vi "SaveData_Roberto.vi"(2 "Quad sub area":dbl format="%#_13g", 4 "Ext time (sec)":dbl=3598463718.5222077 format="%#_10g", 6 "Array":dbl[](array[numeric])=[213.0, 0.002, 401.0, 60.0, 24.0, 3.279, 1.868, 1.4806, 8.203, -0.16493333333333543, 1.0, 1000.0, 1.0, 1.0, 0.0, 0.0101, 0.0101, 0.0101, 0.0099, 0.0101, 0.0099, 0.0099, 0.0099, 0.0099, 0.0098, 0.0098, 0.0098, 0.0096, 0.0096, 0.0096, 0.0095, 0.0095, 0.0095, 0.0093, 0.0093, 0.0093, 0.0093, 0.0092, 0.0092, 0.0092, 0.0092, 0.009, 0.0092, 0.009, 0.009, 0.0089, 0.0089, 0.0089, 0.0089, 0.0087, 0.0087, 0.0087, 0.0087, 0.0087, 0.0085, 0.0087, 0.0085, 0.0084, 0.0085, 0.0085, 0.0084, 0.0082, 0.0082, 0.0082, 0.0081, 0.0081, 0.0081, 0.0081, 0.0081, 0.0081, 0.0079, 0.0079, 0.0079, 0.0079, 0.0078, 0.0078, 0.0076, 0.0076, 0.0076, 0.0078, 0.0078, 0.0078, 0.0076, 0.0075, 0.0075, 0.0075, 0.0073, 0.0075, 0.0075, 0.0073, 0.0073, 0.0073, 0.0072, 0.0072, 0.0072, 0.0072, 0.0072, 0.007, 0.0072, 0.0072, 0.0072, 0.0072, 0.007, 0.007, 0.007, 0.007, 0.0069, 0.0069, 0.0069, 0.007, 0.0069, 0.0069, 0.0067, 0.0069, 0.0069, 0.0067, 0.0067, 0.0069, 0.0067, 0.0066, 0.0066, 0.0066, 0.0066, 0.0067, 0.0066, 0.0066, 0.0066, 0.0066, 0.0066, 0.0066, 0.0064, 0.0064, 0.0064, 0.0066, 0.0064, 0.0064, 0.0066, 0.0064, 0.0064, 0.0064, 0.0066, 0.0066, 0.0064, 0.0064, 0.0064, 0.0064, 0.0064, 0.0064, 0.0064, 0.0064, 0.0066, 0.0066, 0.0064, 0.0066, 0.0066, 0.0066, 0.0066, 0.0066, 0.0066, 0.0064, 0.0067, 0.0067, 0.0067, 0.0069, 0.0069, 0.0069, 0.0072, 0.0072, 0.0073, 0.0073, 0.0073, 0.0075, 0.0076, 0.0078, 0.0079, 0.0082, 0.0084, 0.0087, 0.009, 0.0093, 0.0095, 0.0098, 0.0104, 0.0107, 0.0111, 0.0114, 0.0117, 0.0121, 0.0122, 0.0122, 0.0122, 0.0124, 0.0121, 0.0117, 0.0114, 0.011, 0.0107, 0.0104, 0.0101, 0.0098, 0.0093, 0.0093, 0.0092, 0.009, 0.0089, 0.0089, 0.0089, 0.0087, 0.0085, 0.0085, 0.0085, 0.0084, 0.0085, 0.0082, 0.0081, 0.0081, 0.0079, 0.0079, 0.0079, 0.0078, 0.0079, 0.0079, 0.0079, 0.0079, 0.0079, 0.0081, 0.0082, 0.0082, 0.0082, 0.0085, 0.0084, 0.0084, 0.0085, 0.0082, 0.0082, 0.0082, 0.0081, 0.0079, 0.0078, 0.0076, 0.0075, 0.0073, 0.0072, 0.007, 0.007, 0.007, 0.0072, 0.007, 0.0072, 0.007, 0.007, 0.007, 0.0069, 0.007, 0.0069, 0.007, 0.007, 0.007, 0.007, 0.0069, 0.0069, 0.0069, 0.0069, 0.0067, 0.0067, 0.0067, 0.0067, 0.0066, 0.0066, 0.0067, 0.0064, 0.0064, 0.0066, 0.0066, 0.0066, 0.0067, 0.0067, 0.0067, 0.0066, 0.0069, 0.0069, 0.0069, 0.0067, 0.0069, 0.0069, 0.007, 0.007, 0.007, 0.007, 0.007, 0.0072, 0.0072, 0.0072, 0.0073, 0.0072, 0.0073, 0.0073, 0.0072, 0.0073, 0.0072, 0.0072, 0.007, 0.0072, 0.0072, 0.0072, 0.0072, 0.0072, 0.0072, 0.007, 0.007, 0.007, 0.0072, 0.0072, 0.0072, 0.0073, 0.0072, 0.0072, 0.0072, 0.0072, 0.0073, 0.0073, 0.0072, 0.0073, 0.0073, 0.0073, 0.0073, 0.0073, 0.0073, 0.0073, 0.0073, 0.0075, 0.0075, 0.0075, 0.0075, 0.0076, 0.0078, 0.0075, 0.0076, 0.0078, 0.0078, 0.0078, 0.0078, 0.0078, 0.0078, 0.0078, 0.0078, 0.0079, 0.0079, 0.0079, 0.0079, 0.0079, 0.0081, 0.0082, 0.0081, 0.0084, 0.0084, 0.0084, 0.0084, 0.0085, 0.0084, 0.0085, 0.0085, 0.0087, 0.0087, 0.0089, 0.0089, 0.0089, 0.0089, 0.0089, 0.0089, 0.009, 0.009, 0.0092, 0.009, 0.0092, 0.0092, 0.0093, 0.0093, 0.0095, 0.0095, 0.0095, 0.0095, 0.0096, 0.0096, 0.0098, 0.0098, 0.0099, 0.0099, 0.0101, 0.0101, 0.0101, 0.0101, 0.0101, 0.0102, 0.0102, 0.0102, 0.0102, 0.0104, 0.0104, 0.0104, 0.0107, 0.0105, 0.0107, 0.0108, 0.0108, 0.0108, 0.0108, 0.011, 0.0111, 0.0111, 0.011, 0.0111, 0.0111, 0.0111, 0.0111, 0.0111]) -> (0 "Frequency":dbl=212.9519, 1 "Area":dbl=0.0007273210385932467 format="%#_5g", 3 "Current time (sec)":dbl=3598463780.505753 format="%#_10g", 5 "ADC value":dbl[](array[numeric])=[0.0, 0.0, 0.0, 0.0, 0.0, 0.0, 0.0, 0.0, 0.0, 0.0, 0.0, 0.0, 0.0, 0.0, 0.0, 0.0, 0.0, 0.0, 0.0, 0.0, 0.0, 0.0, 0.0, 0.0, 0.0, 0.0, -0.0, 0.0, 0.0, 0.0, 0.0, -0.0, -0.0, 0.0, 0.0, 0.0, -0.0, 0.0, 0.0, 0.0, 0.0, -0.0, -0.0001, 0.0, 0.0, -0.0, -0.0, -0.0, -0.0, -0.0, -0.0001, -0.0, -0.0, -0.0, 0.0, 0.0, 0.0, 0.0, 0.0, -0.0, -0.0, -0.0, -0.0, -0.0, 0.0, 0.0, 0.0, 0.0, 0.0, -0.0, -0.0, -0.0, 0.0, -0.0, -0.0, -0.0, 0.0, -0.0, -0.0, 0.0, 0.0, 0.0001, 0.0001, 0.0001, 0.0001, 0.0, 0.0001, 0.0, 0.0001, 0.0001, 0.0001, 0.0001, 0.0001, 0.0001, 0.0001, 0.0001, 0.0001, 0.0001, 0.0001, 0.0001, 0.0001, 0.0001, 0.0001, 0.0001, 0.0001, 0.0001, 0.0001, 0.0001, 0.0001, 0.0002, 0.0001, 0.0002, 0.0002, 0.0002, 0.0002, 0.0002, 0.0002, 0.0001, 0.0002, 0.0002, 0.0002, 0.0003, 0.0003, 0.0003, 0.0002, 0.0004, 0.0003, 0.0003, 0.0003, 0.0003, 0.0003, 0.0004, 0.0004, 0.0004, 0.0004, 0.0005, 0.0005, 0.0005, 0.0005, 0.0006, 0.0006, 0.0007, 0.0007, 0.0007, 0.0007, 0.0008, 0.0008, 0.0009, 0.0009, 0.001, 0.0011, 0.0011, 0.0012, 0.0013, 0.0013, 0.0014, 0.0016, 0.0017, 0.0018, 0.0019, 0.0021, 0.0023, 0.0025, 0.0027, 0.0029, 0.0032, 0.0035, 0.0038, 0.0041, 0.0044, 0.0047, 0.005, 0.0052, 0.0053, 0.0054, 0.0054, 0.0053, 0.0052, 0.0049, 0.0047, 0.0044, 0.0041, 0.0038, 0.0036, 0.0034, 0.0031, 0.003, 0.0029, 0.0028, 0.0027, 0.0027, 0.0026, 0.0026, 0.0025, 0.0025, 0.0024, 0.0023, 0.0023, 0.0022, 0.0022, 0.0021, 0.002, 0.002, 0.0019, 0.002, 0.0019, 0.002, 0.002, 0.0021, 0.0021, 0.0021, 0.0023, 0.0023, 0.0023, 0.0024, 0.0024, 0.0024, 0.0024, 0.0023, 0.0022, 0.0022, 0.0021, 0.0019, 0.0018, 0.0017, 0.0016, 0.0015, 0.0014, 0.0013, 0.0013, 0.0013, 0.0012, 0.0012, 0.0012, 0.0012, 0.0012, 0.0012, 0.0011, 0.0011, 0.0011, 0.0012, 0.0011, 0.0011, 0.0011, 0.0011, 0.001, 0.001, 0.001, 0.0009, 0.0008, 0.0008, 0.0007, 0.0007, 0.0006, 0.0007, 0.0006, 0.0006, 0.0006, 0.0006, 0.0006, 0.0005, 0.0005, 0.0006, 0.0006, 0.0006, 0.0006, 0.0006, 0.0006, 0.0007, 0.0007, 0.0007, 0.0007, 0.0007, 0.0007, 0.0007, 0.0008, 0.0008, 0.0008, 0.0008, 0.0008, 0.0008, 0.0007, 0.0007, 0.0007, 0.0006, 0.0006, 0.0006, 0.0006, 0.0005, 0.0005, 0.0004, 0.0005, 0.0004, 0.0003, 0.0003, 0.0003, 0.0003, 0.0003, 0.0003, 0.0003, 0.0003, 0.0003, 0.0003, 0.0002, 0.0002, 0.0002, 0.0002, 0.0002, 0.0002, 0.0001, 0.0001, 0.0001, 0.0002, 0.0001, 0.0001, 0.0001, 0.0001, 0.0, 0.0, -0.0, 0.0001, -0.0, -0.0, 0.0, -0.0, -0.0001, -0.0, -0.0001, -0.0001, -0.0001, -0.0002, -0.0001, -0.0001, -0.0001, -0.0001, -0.0001, -0.0001, -0.0001, -0.0001, -0.0001, -0.0, -0.0, -0.0001, -0.0, -0.0, -0.0, 0.0, 0.0001, 0.0, 0.0, 0.0001, 0.0001, 0.0, 0.0, 0.0, -0.0, -0.0, -0.0, -0.0001, -0.0, -0.0, -0.0, -0.0001, -0.0, -0.0, -0.0, -0.0, -0.0, 0.0, 0.0, 0.0, 0.0, 0.0001, 0.0, 0.0, 0.0, 0.0, 0.0, 0.0, 0.0, 0.0, 0.0, 0.0, 0.0, 0.0, 0.0, 0.0, 0.0, 0.0, 0.0, 0.0, 0.0, 0.0, 0.0, 0.0, 0.0, 0.0, 0.0, 0.0, 0.0, 0.0])   [LabVIEW 2018]
uses:
  Global 2.vi
  kleinjan/MKS/Global - Pressure & Flow.vi
  <vilib>/Utility/file.llb/Write To Spreadsheet File (string).vi
  <vilib>/Utility/file.llb/Write To Spreadsheet File (DBL).vi
panel:
  out "Fit OK":bool=TRUE
  out "Fupper":dbl=213.3 format="%#_13g"
  out "Flower":dbl=212.75 format="%#_13g"
  out "Python data":i32=2914
  out "String to python":string="213 MHz crystal, SMT03 RF Gen\r\nQCV3598374279.csv\r\nUnused\r\nNMRave.csv\r\nUnused\r\nTune2.csv\r\n\r\n\r\n  212.7500\r\n  213.3000\r\n35984.0000\r\n63780.5058\r\n  213.0000\r\n    0.0020\r\n  401.0000\r\n   60.0000\r\n   24.0000\r\n    3.2790\r\n    1.8680\r\n    1.4806\r\n    8.2030\r\n   -0.1649\r\n    1.0000\r\n 1000.0000\r\n    1.0000\r\n    1.0000\r\n    0.0000\r\n    4.0771\r\n    2.0000\r\n  212.9500\r\n    0.0000\r\n    0.0000\r\n    4.0000\r\n    2.1333\r\n   33.8900\r\n    0.0101\r\n    0.0101\r\n    0.0101\r\n    0.0099\r\n    0.0101\r\n    0.0099\r\n    0.0099\r\n    0.0099\r\n    0.0099\r\n    0.0098\r\n    0.0098\r\n    0.0098\r\n    0.0096\r\n    0.0096\r\n    0.0096\r\n    0.0095\r\n    0.0095\r\n    0.0095\r\n    0.0093\r\n    0.0093\r\n    0.0093\r\n    0.0093\r\n    0.0092\r\n    0.0092\r\n    0.0092\r\n    0.0092\r\n    0.0090\r\n    0.0092\r\n    0.0090\r\n    0.0090\r\n    0.0089\r\n    0.0089\r\n    0.0089\r\n    0.0089\r\n    0.0087\r\n    0.0087\r\n    0.0087\r\n    0.0087\r\n    0.0087\r\n    0.0085\r\n    0.0087\r\n    0.0085\r\n    0.0084\r\n    0.0085\r\n    0.0085\r\n    0.0084\r\n    0.0082\r\n    0.0082\r\n    0.0082\r\n    0.0081\r\n    0.0081\r\n    0.0081\r\n    0.0081\r\n    0.0081\r\n    0.0081\r\n    0.0079\r\n    0.0079\r\n    0.0079\r\n    0.0079\r\n    0.0078\r\n    0.0078\r\n    0.0076\r\n    0.0076\r\n    0.0076\r\n    0.0078\r\n    0.0078\r\n    0.0078\r\n    0.0076\r\n    0.0075\r\n    0.0075\r\n    0.0075\r\n    0.0073\r\n    0.0075\r\n    0.0075\r\n    0.0073\r\n    0.0073\r\n    0.0073\r\n    0.0072\r\n    0.0072\r\n    0.0072\r\n    0.0072\r\n    0.0072\r\n    0.0070\r\n    0.0072\r\n    0.0072\r\n    0.0072\r\n    0.0072\r\n    0.0070\r\n    0.0070\r\n    0.0070\r\n    0.0070\r\n    0.0069\r\n    0.0069\r\n    0.0069\r\n    0.0070\r\n    0.0069\r\n    0.0069\r\n    0.0067\r\n    0.0069\r\n    0.0069\r\n    0.0067\r\n    0.0067\r\n    0.0069\r\n    0.0067\r\n    0.0066\r\n    0.0066\r\n    0.0066\r\n    0.0066\r\n    0.0067\r\n    0.0066\r\n    0.0066\r\n    0.0066\r\n    0.0066\r\n    0.0066\r\n    0.0066\r\n    0.0064\r\n    0.0064\r\n    0.0064\r\n    0.0066\r\n    0.0064\r\n    0.0064\r\n    0.0066\r\n    0.0064\r\n    0.0064\r\n    0.0064\r\n    0.0066\r\n    0.0066\r\n    0.0064\r\n    0.0064\r\n    0.0064\r\n    0.0064\r\n    0.0064\r\n    0.0064\r\n    0.0064\r\n    0.0064\r\n    0.0066\r\n    0.0066\r\n    0.0064\r\n    0.0066\r\n    0.0066\r\n    0.0066\r\n    0.0066\r\n    0.0066\r\n    0.0066\r\n    0.0064\r\n    0.0067\r\n    0.0067\r\n    0.0067\r\n    0.0069\r\n    0.0069\r\n    0.0069\r\n    0.0072\r\n    0.0072\r\n    0.0073\r\n    0.0073\r\n    0.0073\r\n    0.0075\r\n    0.0076\r\n    0.0078\r\n    0.0079\r\n    0.0082\r\n    0.0084\r\n    0.0087\r\n    0.0090\r\n    0.0093\r\n    0.0095\r\n    0.0098\r\n    0.0104\r\n    0.0107\r\n    0.0111\r\n    0.0114\r\n    0.0117\r\n    0.0121\r\n    0.0122\r\n    0.0122\r\n    0.0122\r\n    0.0124\r\n    0.0121\r\n    0.0117\r\n    0.0114\r\n    0.0110\r\n    0.0107\r\n    0.0104\r\n    0.0101\r\n    0.0098\r\n    0.0093\r\n    0.0093\r\n    0.0092\r\n    0.0090\r\n    0.0089\r\n    0.0089\r\n    0.0089\r\n    0.0087\r\n    0.0085\r\n    0.0085\r\n    0.0085\r\n    0.0084\r\n    0.0085\r\n    0.0082\r\n    0.0081\r\n    0.0081\r\n    0.0079\r\n    0.0079\r\n    0.0079\r\n    0.0078\r\n    0.0079\r\n    0.0079\r\n    0.0079\r\n    0.0079\r\n    0.0079\r\n    0.0081\r\n    0.0082\r\n    0.0082\r\n    0.0082\r\n    0.0085\r\n    0.0084\r\n    0.0084\r\n    0.0085\r\n    0.0082\r\n    0.0082\r\n    0.0082\r\n    0.0081\r\n    0.0079\r\n    0.0078\r\n    0.0076\r\n    0.0075\r\n    0.0073\r\n    0.0072\r\n    0.0070\r\n    0.0070\r\n    0.0070\r\n    0.0072\r\n    0.0070\r\n    0.0072\r\n    0.0070\r\n    0.0070\r\n    0.0070\r\n    0.0069\r\n    0.0070\r\n    0.0069\r\n    0.0070\r\n    0.0070\r\n    0.0070\r\n    0.0070\r\n    0.0069\r\n    0.0069\r\n    0.0069\r\n    0.0069\r\n    0.0067\r\n    0.0067\r\n    0.0067\r\n    0.0067\r\n    0.0066\r\n    0.0066\r\n    0.0067\r\n    0.0064\r\n    0.0064\r\n    0.0066\r\n    0.0066\r\n    0.0066\r\n    0.0067\r\n    0.0067\r\n    0.0067\r\n    0.0066\r\n    0.0069\r\n    0.0069\r\n    0.0069\r\n    0.0067\r\n    0.0069\r\n    0.0069\r\n    0.0070\r\n    0.0070\r\n    0.0070\r\n    0.0070\r\n    0.0070\r\n    0.0072\r\n    0.0072\r\n    0.0072\r\n    0.0073\r\n    0.0072\r\n    0.0073\r\n    0.0073\r\n    0.0072\r\n    0.0073\r\n    0.0072\r\n    0.0072\r\n    0.0070\r\n    0.0072\r\n    0.0072\r\n    0.0072\r\n    0.0072\r\n    0.0072\r\n    0.0072\r\n    0.0070\r\n    0.0070\r\n    0.0070\r\n    0.0072\r\n    0.0072\r\n    0.0072\r\n    0.0073\r\n    0.0072\r\n    0.0072\r\n    0.0072\r\n    0.0072\r\n    0.0073\r\n    0.0073\r\n    0.0072\r\n    0.0073\r\n    0.0073\r\n    0.0073\r\n    0.0073\r\n    0.0073\r\n    0.0073\r\n    0.0073\r\n    0.0073\r\n    0.0075\r\n    0.0075\r\n    0.0075\r\n    0.0075\r\n    0.0076\r\n    0.0078\r\n    0.0075\r\n    0.0076\r\n    0.0078\r\n    0.0078\r\n    0.0078\r\n    0.0078\r\n    0.0078\r\n    0.0078\r\n    0.0078\r\n    0.0078\r\n    0.0079\r\n    0.0079\r\n    0.0079\r\n    0.0079\r\n    0.0079\r\n    0.0081\r\n    0.0082\r\n    0.0081\r\n    0.0084\r\n    0.0084\r\n    0.0084\r\n    0.0084\r\n    0.0085\r\n    0.0084\r\n    0.0085\r\n    0.0085\r\n    0.0087\r\n    0.0087\r\n    0.0089\r\n    0.0089\r\n    0.0089\r\n    0.0089\r\n    0.0089\r\n    0.0089\r\n    0.0090\r\n    0.0090\r\n    0.0092\r\n    0.0090\r\n    0.0092\r\n    0.0092\r\n    0.0093\r\n    0.0093\r\n    0.0095\r\n    0.0095\r\n    0.0095\r\n    0.0095\r\n    0.0096\r\n    0.0096\r\n    0.0098\r\n    0.0098\r\n    0.0099\r\n    0.0099\r\n    0.0101\r\n    0.0101\r\n    0.0101\r\n    0.0101\r\n    0.0101\r\n    0.0102\r\n    0.0102\r\n    0.0102\r\n    0.0102\r\n    0.0104\r\n    0.0104\r\n    0.0104\r\n    0.0107\r\n    0.0105\r\n    0.0107\r\n    0.0108\r\n    0.0108\r\n    0.0108\r\n    0.0108\r\n    0.0110\r\n    0.0111\r\n    0.0111\r\n    0.0110\r\n    0.0111\r\n    0.0111\r\n    0.0111\r\n    0.0111\r\n    0.0111\r\n?"
  out "Amplitude":dbl=0.0069 format="%#_5g"
  out "ADC Voltage Chart":dbl(graph)
  out "String from python":string="1\n212.9519\n0.0069\n0.0007273210385932467\n0.0000\n0.0000\n0.0000\n0.0000\n0.0000\n0.0000\n0.0000\n0.0000\n0.0000\n0.0000\n0.0000\n0.0000\n0.0000\n0.0000\n0.0000\n0.0000\n0.0000\n0.0000\n0.0000\n0.0000\n0.0000\n0.0000\n0.0000\n0.0000\n0.0000\n0.0000\n-0.0000\n0.0000\n0.0000\n0.0000\n0.0000\n-0.0000\n-0.0000\n0.0000\n0.0000\n0.0000\n-0.0000\n0.0000\n0.0000\n0.0000\n0.0000\n-0.0000\n-0.0001\n0.0000\n0.0000\n-0.0000\n-0.0000\n-0.0000\n-0.0000\n-0.0000\n-0.0001\n-0.0000\n-0.0000\n-0.0000\n0.0000\n0.0000\n0.0000\n0.0000\n0.0000\n-0.0000\n-0.0000\n-0.0000\n-0.0000\n-0.0000\n0.0000\n0.0000\n0.0000\n0.0000\n0.0000\n-0.0000\n-0.0000\n-0.0000\n0.0000\n-0.0000\n-0.0000\n-0.0000\n0.0000\n-0.0000\n-0.0000\n0.0000\n0.0000\n0.0001\n0.0001\n0.0001\n0.0001\n0.0000\n0.0001\n0.0000\n0.0001\n0.0001\n0.0001\n0.0001\n0.0001\n0.0001\n0.0001\n0.0001\n0.0001\n0.0001\n0.0001\n0.0001\n0.0001\n0.0001\n0.0001\n0.0001\n0.0001\n0.0001\n0.0001\n0.0001\n0.0001\n0.0002\n0.0001\n0.0002\n0.0002\n0.0002\n0.0002\n0.0002\n0.0002\n0.0001\n0.0002\n0.0002\n0.0002\n0.0003\n0.0003\n0.0003\n0.0002\n0.0004\n0.0003\n0.0003\n0.0003\n0.0003\n0.0003\n0.0004\n0.0004\n0.0004\n0.0004\n0.0005\n0.0005\n0.0005\n0.0005\n0.0006\n0.0006\n0.0007\n0.0007\n0.0007\n0.0007\n0.0008\n0.0008\n0.0009\n0.0009\n0.0010\n0.0011\n0.0011\n0.0012\n0.0013\n0.0013\n0.0014\n0.0016\n0.0017\n0.0018\n0.0019\n0.0021\n0.0023\n0.0025\n0.0027\n0.0029\n0.0032\n0.0035\n0.0038\n0.0041\n0.0044\n0.0047\n0.0050\n0.0052\n0.0053\n0.0054\n0.0054\n0.0053\n0.0052\n0.0049\n0.0047\n0.0044\n0.0041\n0.0038\n0.0036\n0.0034\n0.0031\n0.0030\n0.0029\n0.0028\n0.0027\n0.0027\n0.0026\n0.0026\n0.0025\n0.0025\n0.0024\n0.0023\n0.0023\n0.0022\n0.0022\n0.0021\n0.0020\n0.0020\n0.0019\n0.0020\n0.0019\n0.0020\n0.0020\n0.0021\n0.0021\n0.0021\n0.0023\n0.0023\n0.0023\n0.0024\n0.0024\n0.0024\n0.0024\n0.0023\n0.0022\n0.0022\n0.0021\n0.0019\n0.0018\n0.0017\n0.0016\n0.0015\n0.0014\n0.0013\n0.0013\n0.0013\n0.0012\n0.0012\n0.0012\n0.0012\n0.0012\n0.0012\n0.0011\n0.0011\n0.0011\n0.0012\n0.0011\n0.0011\n0.0011\n0.0011\n0.0010\n0.0010\n0.0010\n0.0009\n0.0008\n0.0008\n0.0007\n0.0007\n0.0006\n0.0007\n0.0006\n0.0006\n0.0006\n0.0006\n0.0006\n0.0005\n0.0005\n0.0006\n0.0006\n0.0006\n0.0006\n0.0006\n0.0006\n0.0007\n0.0007\n0.0007\n0.0007\n0.0007\n0.0007\n0.0007\n0.0008\n0.0008\n0.0008\n0.0008\n0.0008\n0.0008\n0.0007\n0.0007\n0.0007\n0.0006\n0.0006\n0.0006\n0.0006\n0.0005\n0.0005\n0.0004\n0.0005\n0.0004\n0.0003\n0.0003\n0.0003\n0.0003\n0.0003\n0.0003\n0.0003\n0.0003\n0.0003\n0.0003\n0.0002\n0.0002\n0.0002\n0.0002\n0.0002\n0.0002\n0.0001\n0.0001\n0.0001\n0.0002\n0.0001\n0.0001\n0.0001\n0.0001\n0.0000\n0.0000\n-0.0000\n0.0001\n-0.0000\n-0.0000\n0.0000\n-0.0000\n-0.0001\n-0.0000\n-0.0001\n-0.0001\n-0.0001\n-0.0002\n-0.0001\n-0.0001\n-0.0001\n-0.0001\n-0.0001\n-0.0001\n-0.0001\n-0.0001\n-0.0001\n-0.0000\n-0.0000\n-0.0001\n-0.0000\n-0.0000\n-0.0000\n0.0000\n0.0001\n0.0000\n0.0000\n0.0001\n0.0001\n0.0000\n0.0000\n0.0000\n-0.0000\n-0.0000\n-0.0000\n-0.0001\n-0.0000\n-0.0000\n-0.0000\n-0.0001\n-0.0000\n-0.0000\n-0.0000\n-0.0000\n-0.0000\n0.0000\n0.0000\n0.0000\n0.0000\n0.0001\n0.0000\n0.0000\n0.0000\n0.0000\n0.0000\n0.0000\n0.0000\n0.0000\n0.0000\n0.0000\n0.0000\n0.0000\n0.0000\n0.0000\n0.0000\n0.0000\n0.0000\n0.0000\n0.0000\n0.0000\n0.0000\n0.0000\n0.0000\n0.0000\n0.0000\n0.0000\n0.0000\n0.0000\n?"
  out "Day":string="10"
  out "Appended array":dbl[](array[numeric])=[35984.0, 63780.505753040314, 213.0, 0.002, 401.0, 60.0, 24.0, 3.279, 1.868, 1.4806, 8.203, -0.16493333333333543, 1.0, 1000.0, 1.0, 1.0, 0.0, 4.077083110809326, 2.0, 212.9499969482422, 0.0, 0.0, 4.0, 2.13326012312, 33.89, 0.0101, 0.0101, 0.0101, 0.0099, 0.0101, 0.0099, 0.0099, 0.0099, 0.0099, 0.0098, 0.0098, 0.0098, 0.0096, 0.0096, 0.0096, 0.0095, 0.0095, 0.0095, 0.0093, 0.0093, 0.0093, 0.0093, 0.0092, 0.0092, 0.0092, 0.0092, 0.009, 0.0092, 0.009, 0.009, 0.0089, 0.0089, 0.0089, 0.0089, 0.0087, 0.0087, 0.0087, 0.0087, 0.0087, 0.0085, 0.0087, 0.0085, 0.0084, 0.0085, 0.0085, 0.0084, 0.0082, 0.0082, 0.0082, 0.0081, 0.0081, 0.0081, 0.0081, 0.0081, 0.0081, 0.0079, 0.0079, 0.0079, 0.0079, 0.0078, 0.0078, 0.0076, 0.0076, 0.0076, 0.0078, 0.0078, 0.0078, 0.0076, 0.0075, 0.0075, 0.0075, 0.0073, 0.0075, 0.0075, 0.0073, 0.0073, 0.0073, 0.0072, 0.0072, 0.0072, 0.0072, 0.0072, 0.007, 0.0072, 0.0072, 0.0072, 0.0072, 0.007, 0.007, 0.007, 0.007, 0.0069, 0.0069, 0.0069, 0.007, 0.0069, 0.0069, 0.0067, 0.0069, 0.0069, 0.0067, 0.0067, 0.0069, 0.0067, 0.0066, 0.0066, 0.0066, 0.0066, 0.0067, 0.0066, 0.0066, 0.0066, 0.0066, 0.0066, 0.0066, 0.0064, 0.0064, 0.0064, 0.0066, 0.0064, 0.0064, 0.0066, 0.0064, 0.0064, 0.0064, 0.0066, 0.0066, 0.0064, 0.0064, 0.0064, 0.0064, 0.0064, 0.0064, 0.0064, 0.0064, 0.0066, 0.0066, 0.0064, 0.0066, 0.0066, 0.0066, 0.0066, 0.0066, 0.0066, 0.0064, 0.0067, 0.0067, 0.0067, 0.0069, 0.0069, 0.0069, 0.0072, 0.0072, 0.0073, 0.0073, 0.0073, 0.0075, 0.0076, 0.0078, 0.0079, 0.0082, 0.0084, 0.0087, 0.009, 0.0093, 0.0095, 0.0098, 0.0104, 0.0107, 0.0111, 0.0114, 0.0117, 0.0121, 0.0122, 0.0122, 0.0122, 0.0124, 0.0121, 0.0117, 0.0114, 0.011, 0.0107, 0.0104, 0.0101, 0.0098, 0.0093, 0.0093, 0.0092, 0.009, 0.0089, 0.0089, 0.0089, 0.0087, 0.0085, 0.0085, 0.0085, 0.0084, 0.0085, 0.0082, 0.0081, 0.0081, 0.0079, 0.0079, 0.0079, 0.0078, 0.0079, 0.0079, 0.0079, 0.0079, 0.0079, 0.0081, 0.0082, 0.0082, 0.0082, 0.0085, 0.0084, 0.0084, 0.0085, 0.0082, 0.0082, 0.0082, 0.0081, 0.0079, 0.0078, 0.0076, 0.0075, 0.0073, 0.0072, 0.007, 0.007, 0.007, 0.0072, 0.007, 0.0072, 0.007, 0.007, 0.007, 0.0069, 0.007, 0.0069, 0.007, 0.007, 0.007, 0.007, 0.0069, 0.0069, 0.0069, 0.0069, 0.0067, 0.0067, 0.0067, 0.0067, 0.0066, 0.0066, 0.0067, 0.0064, 0.0064, 0.0066, 0.0066, 0.0066, 0.0067, 0.0067, 0.0067, 0.0066, 0.0069, 0.0069, 0.0069, 0.0067, 0.0069, 0.0069, 0.007, 0.007, 0.007, 0.007, 0.007, 0.0072, 0.0072, 0.0072, 0.0073, 0.0072, 0.0073, 0.0073, 0.0072, 0.0073, 0.0072, 0.0072, 0.007, 0.0072, 0.0072, 0.0072, 0.0072, 0.0072, 0.0072, 0.007, 0.007, 0.007, 0.0072, 0.0072, 0.0072, 0.0073, 0.0072, 0.0072, 0.0072, 0.0072, 0.0073, 0.0073, 0.0072, 0.0073, 0.0073, 0.0073, 0.0073, 0.0073, 0.0073, 0.0073, 0.0073, 0.0075, 0.0075, 0.0075, 0.0075, 0.0076, 0.0078, 0.0075, 0.0076, 0.0078, 0.0078, 0.0078, 0.0078, 0.0078, 0.0078, 0.0078, 0.0078, 0.0079, 0.0079, 0.0079, 0.0079, 0.0079, 0.0081, 0.0082, 0.0081, 0.0084, 0.0084, 0.0084, 0.0084, 0.0085, 0.0084, 0.0085, 0.0085, 0.0087, 0.0087, 0.0089, 0.0089, 0.0089, 0.0089, 0.0089, 0.0089, 0.009, 0.009, 0.0092, 0.009, 0.0092, 0.0092, 0.0093, 0.0093, 0.0095, 0.0095, 0.0095, 0.0095, 0.0096, 0.0096, 0.0098, 0.0098, 0.0099, 0.0099, 0.0101, 0.0101, 0.0101, 0.0101, 0.0101, 0.0102, 0.0102, 0.0102, 0.0102, 0.0104, 0.0104, 0.0104, 0.0107, 0.0105, 0.0107, 0.0108, 0.0108, 0.0108, 0.0108, 0.011, 0.0111, 0.0111, 0.011, 0.0111, 0.0111, 0.0111, 0.0111, 0.0111] format="%#_10g"
  out "File name":string="C:\\users\\plm\\Desktop\\rssmt\\data\\10\\QCV3598463719.csv"
  in  "Save Data to File":bool=TRUE
  # "Saves data to spreadsheet file"
  # "Creates file with name including current time\nand header plus data"
  # "NMR signal Edges (MHz)"
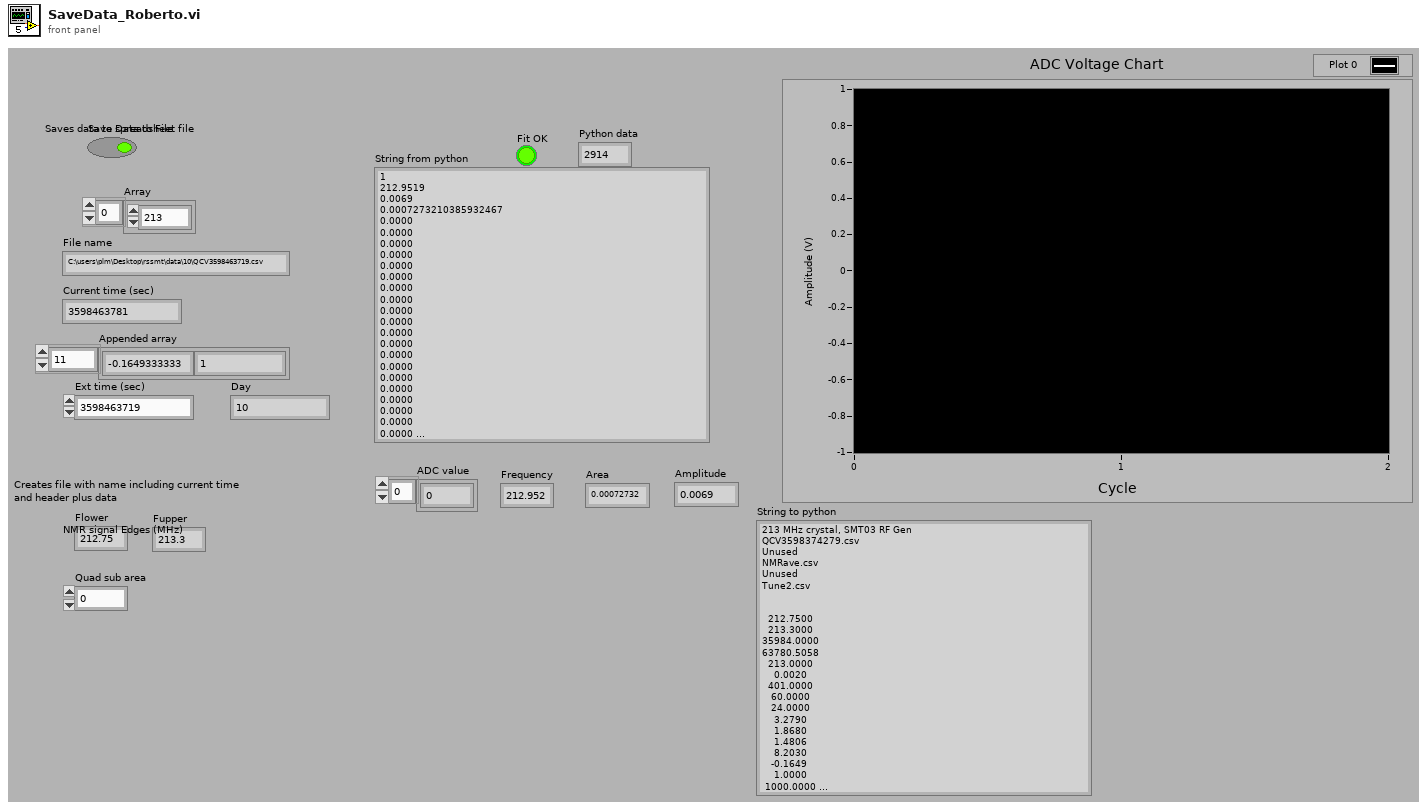
[diagram p1: front panel]
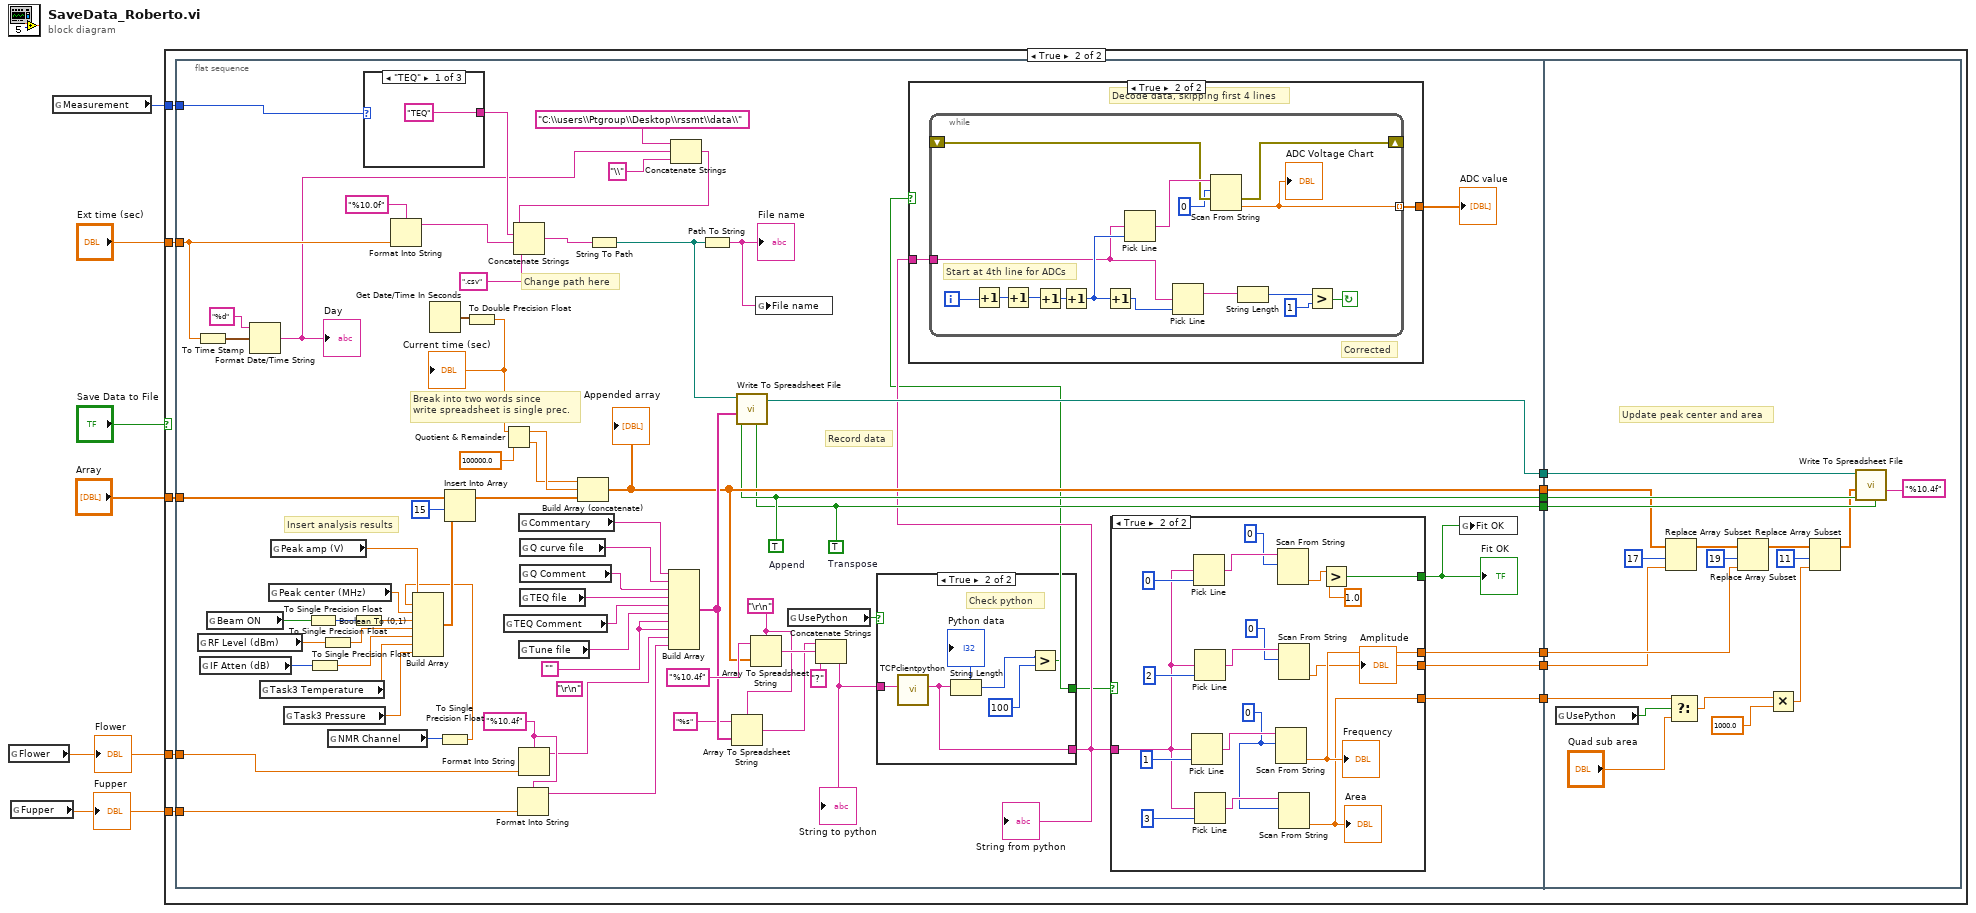
[diagram p0: block diagram]
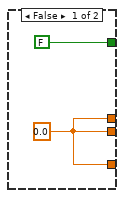
[diagram p4: hidden frame]
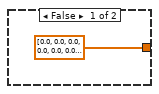
[diagram p5: hidden frame]
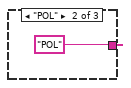
[diagram p6: hidden frame]
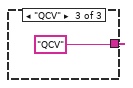
[diagram p7: hidden frame]
diagram:
  n1 = global read "Global 2.vi" "Flower"() -> (w2:dbl)
  "Flower" <- w2
  n2 = global read "Global 2.vi" "Fupper"() -> (w1:dbl)
  "Fupper" <- w1
  n3 = global read "Global 2.vi" "Measurement"() -> (w3:enum16{"TEQ", "POL", "QCV"})
  n4 = case shown="True" "Save Data to File" {
    tunnel: "Array" -> [_ w17]
    tunnel: "Ext time (sec)" -> [_ w16]
    tunnel: w3 -> [_ w18]
    tunnel: w2 -> [_ w8]
    tunnel: w1 -> [_ w7]
    frame False {
      # "Not writing file"
    }
    frame True {
      n5 = flat-sequence {
        tunnel: w18 -> [w76]
        tunnel: w17 -> [w72]
        tunnel: w16 -> [w54]
        tunnel: [w37] -> w15
        tunnel: [w36] -> w14
        tunnel: [w35] -> w13
        tunnel: [w34] -> w12
        tunnel: [w33] -> w11
        tunnel: [w32] -> w10
        tunnel: [w31] -> w9
        tunnel: w8 -> [w27]
        tunnel: w7 -> [w28]
        tunnel: w15 -> [w149]
        tunnel: w14 -> [w140]
        tunnel: w13 -> [w154]
        tunnel: w12 -> [w142]
        tunnel: w11 -> [w153]
        tunnel: w10 -> [w152]
        tunnel: w9 -> [w143]
        frame #0 {
          w26 = "%10.4f"
          (unwired) "\r\n"
          w40 = "\r\n"
          w66 = ""
          w33 = TRUE  # Append
          w32 = TRUE  # Transpose
          # "Insert analysis results"
          # "Change path here"
          # "Record data"
          # "Break into two words since\nwrite spreadsheet is single prec."
          n6 = To Time Stamp(1:w54) -> (0:w53:timestamp)
          n7 = global read "Global 2.vi" "RF Level (dBm)"() -> (w60:dbl)
          n8 = global read "Global 2.vi" "IF Atten (dB)"() -> (w58:i8)
          n9 = global read "Global 2.vi" "Beam ON"() -> (w62:bool)
          n10 = Format Date/Time String(time format string (%c)="%d", seconds (now)=w53) -> (date/time string=w50:string)  [unwired: 1 in]
          "Day" <- w50
          n11 = global read "Global - Pressure & Flow.vi" "Task3 Temperature"() -> (w56:dbl)
          n12 = global read "Global 2.vi" "Peak center (MHz)"() -> (w67:sgl)
          n13 = global read "Global 2.vi" "Peak amp (V)"() -> (w69:sgl)
          n14 = global read "Global - Pressure & Flow.vi" "Task3 Pressure"() -> (w55:dbl)
          n15 = Boolean To (0,1)(Boolean=w62) -> (0, 1=w63:i16)
          n16 = To Single Precision Float(number=w58) -> (single precision float=w57:sgl)
          n17 = To Single Precision Float(number=w60) -> (single precision float=w59:sgl)
          n18 = global read "Global 2.vi" "NMR Channel"() -> (w65:i32)
          n19 = To Single Precision Float(number=w63) -> (single precision float=w61:sgl)
          n20 = case shown="\"TEQ\"" w76 {
            tunnel: ["TEQ" "POL" "QCV"] -> w75
            frame "TEQ" {
            }
            frame "POL" {
            }
            frame "QCV" {
            }
          }
          n21 = Format Into String "Format Into String"(format string="%10.0f", w54) -> (resulting string=w86:string)  [unwired: 2 in, 1 out]
          n22 = Get Date/Time In Seconds() -> (seconds since 1Jan1904=w83:timestamp)
          n23 = To Single Precision Float(number=w65) -> (single precision float=w64:sgl)
          n24 = Build Array(w69, w64, w67, w61, w59, w57, w56, w55) -> (w68:dbl[])
          n25 = Insert Into Array "Insert Into Array"(array=w72, index=15, new element=w68) -> (w71:dbl[])
          n26 = To Double Precision Float(number=w83) -> (double precision float=w82:dbl)
          "Current time (sec)" <- w82
          n27 = Quotient & Remainder(x=w82, y=100000.0) -> (x-y*floor(x/y)=w81:dbl, floor(x/y)=w79:dbl)
          n28 = global read "Global 2.vi" "TEQ Comment"() -> (w74:string)
          n29 = Format Into String(format string=w26, w28) -> (resulting string=w24:string)  [unwired: 2 in, 1 out]
          n30 = global read "Global 2.vi" "Commentary"() -> (w44:string)
          n31 = global read "Global 2.vi" "Tune file"() -> (w47:string)
          n32 = Format Into String(format string=w26, w27) -> (resulting string=w25:string)  [unwired: 2 in, 1 out]
          n33 = global read "Global 2.vi" "Q curve file"() -> (w43:string)
          n34 = global read "Global 2.vi" "Q Comment"() -> (w42:string)
          n35 = global read "Global 2.vi" "TEQ file"() -> (w73:string)
          n36 = Build Array (concatenate) "Build Array"(w79, w81, w71) -> (w34:dbl[])
          "Appended array" <- w34
          n37 = Build Array(w44, w43, w42, w73, w74, w47, w66, w66, w25, w24) -> (w41:string[])
          n38 = Concatenate Strings("C:\\users\\Ptgroup\\Desktop\\rssmt\\data\\", w50, "\\") -> (w48:string)
          n39 = Concatenate Strings(w48, w75, w86, ".csv") -> (w84:string)
          n40 = String To Path(string=w84) -> (path=w77:path)
          n41 = Path To String(path=w77) -> (string=w78:string)
          "File name" <- w78
          n42 = Array To Spreadsheet String(delimiter (Tab)=w40, array=w41, 3:"%s") -> (spreadsheet string=w39:string)
          n43 = call-poly <vilib>:"Write To Spreadsheet File.vi"("transpose? (no:F)"=w32, "append to file? (new file:F)"=w33, "1D data"=w41, "file path (dialog if empty)"=w77) -> ("new file path (Not A Path if cancelled)"=w35:path)  [unwired: 4 in]
          n44 = Array To Spreadsheet String(delimiter (Tab)=w40, array=w34, 3:"%10.4f") -> (spreadsheet string=w45:string)
          n45 = global write "Global 2.vi" "File name"(w78) -> ()
          n46 = global read "Global 2.vi" "UsePython"() -> (w19:bool)
          n47 = Concatenate Strings(w39, w45, "?") -> (w29:string)
          "String to python" <- w29
          n48 = case shown="True" w19 {
            selector: w19 -> [w89 _]
            tunnel: w29 -> [w88 w94]
            tunnel: [w88 w93] -> w23
            tunnel: [w89 w90] -> w21
            frame False {
            }
            frame True {
              # "Check python"
              n49 = call "TCPclientpython.vi"("Input Command"=w94) -> ("Command and Results"=w93:string)  [unwired: 4 in, 2 out]
              n50 = String Length(string=w93) -> (length=w91:i32)
              "Python data" <- w91
              n51 = Greater?(x=w91, y=100) -> (0:w90:bool)
            }
          }
          "String from python" <- w23
          n52 = case shown="True" w21 {
            tunnel: w23 -> [_ w117]
            tunnel: [dbl[] [0.0, 0.0, 0.0, 0.0, 0.0, 0.0, 0.0, 0.0, 0.0, 0.0, 0.0, 0.0, 0.0, 0.0, 0.0, 0.0, 0.0, 0.0, 0.0, 0.0, 0.0, 0.0, 0.0, 0.0, 0.0, 0.0, 0.0001, 0.0001, 0.0001, 0.0, -0.0, -0.0, -0.0, -0.0001, -0.0001, -0.0001, -0.0, -0.0001, -0.0, 0.0, 0.0, 0.0, 0.0, -0.0, 0.0, -0.0, -0.0001, -0.0, -0.0, -0.0001, -0.0001, -0.0001, -0.0, -0.0001, -0.0, 0.0, 0.0001, 0.0001, 0.0001, 0.0001, 0.0001, 0.0001, 0.0001, 0.0001, 0.0, -0.0, -0.0, -0.0, -0.0, -0.0, -0.0, 0.0, 0.0, 0.0, 0.0, 0.0001, 0.0002, 0.0001, 0.0001, 0.0001, 0.0001, 0.0001, 0.0, 0.0, 0.0, 0.0, 0.0, 0.0, 0.0, 0.0, 0.0, 0.0001, 0.0001, 0.0001, 0.0001, 0.0001, 0.0001, 0.0001, 0.0001, -0.0, -0.0, 0.0, -0.0001, -0.0001, -0.0001, -0.0001, -0.0001, -0.0, 0.0, -0.0, 0.0, 0.0001, 0.0, 0.0, 0.0, 0.0, -0.0, -0.0001, -0.0001, -0.0001, -0.0001, -0.0001, -0.0001, -0.0001, -0.0001, -0.0001, -0.0, -0.0, -0.0, 0.0, 0.0, 0.0, 0.0, -0.0, 0.0, -0.0, -0.0001, -0.0001, -0.0001, -0.0001, -0.0001, -0.0001, -0.0, 0.0, 0.0, 0.0, 0.0, -0.0, 0.0, -0.0, -0.0001, -0.0001, -0.0001, -0.0002, -0.0002, -0.0002, -0.0002, -0.0002, -0.0001, -0.0002, -0.0001, -0.0001, -0.0001, -0.0, -0.0001, -0.0, -0.0001, -0.0002, -0.0002, -0.0002, -0.0002, -0.0002, -0.0003, -0.0003, -0.0003, -0.0003, -0.0003, -0.0004, -0.0003, -0.0003, -0.0002, -0.0002, -0.0002, -0.0002, -0.0002, -0.0002, -0.0002, -0.0002, -0.0002, -0.0002, -0.0002, -0.0003, -0.0003, -0.0002, -0.0002, -0.0002, -0.0002, -0.0001, -0.0001, -0.0001, -0.0001, -0.0001, -0.0001, -0.0001, -0.0002, -0.0002, -0.0001, -0.0001, -0.0002, -0.0002, -0.0002, -0.0002, -0.0002, -0.0002, -0.0002, -0.0002, -0.0002, -0.0002, -0.0002, -0.0002, -0.0002, -0.0002, -0.0002, -0.0002, -0.0002, -0.0002, -0.0002, -0.0002, -0.0002, -0.0002, -0.0001, -0.0001, -0.0001, -0.0, -0.0001, -0.0001, -0.0001, -0.0001, -0.0001, -0.0001, -0.0001, -0.0002, -0.0002, -0.0002, -0.0002, -0.0003, -0.0002, -0.0002, -0.0001, -0.0001, -0.0, -0.0, -0.0, -0.0001, -0.0001, -0.0001, -0.0001, -0.0001, -0.0001, -0.0001, -0.0001, -0.0002, -0.0002, -0.0002, -0.0001, -0.0001, -0.0001, -0.0001, -0.0001, 0.0, -0.0, -0.0, -0.0001, -0.0001, -0.0, -0.0001, -0.0001, -0.0001, -0.0002, -0.0002, -0.0001, -0.0001, -0.0001, -0.0001, -0.0001, -0.0001, -0.0, -0.0001, -0.0001, -0.0, -0.0001, -0.0001, -0.0001, -0.0001, -0.0001, -0.0001, -0.0001, -0.0002, -0.0001, -0.0001, -0.0001, -0.0002, -0.0001, -0.0001, -0.0001, -0.0001, -0.0, -0.0, -0.0001, -0.0001, -0.0001, -0.0001, -0.0001, -0.0001, -0.0001, -0.0001, -0.0001, -0.0001, -0.0001, -0.0, -0.0, 0.0, -0.0, 0.0, 0.0, 0.0, 0.0, -0.0, 0.0, 0.0, -0.0001, -0.0001, -0.0001, -0.0001, -0.0, -0.0, -0.0, 0.0, 0.0001, 0.0001, 0.0001, 0.0001, 0.0001, 0.0001, 0.0, -0.0, -0.0, -0.0, -0.0, -0.0, -0.0, 0.0, 0.0, 0.0, -0.0, 0.0001, 0.0, 0.0, 0.0, 0.0001, 0.0, 0.0, 0.0001, 0.0, -0.0, -0.0001, -0.0001, -0.0, -0.0001, 0.0, -0.0001, -0.0, -0.0, 0.0, 0.0001, 0.0, 0.0, 0.0, 0.0, 0.0, 0.0, 0.0, 0.0, 0.0, 0.0, 0.0, 0.0, 0.0, 0.0, 0.0, 0.0, 0.0, 0.0, 0.0, 0.0, 0.0, 0.0, 0.0, 0.0, 0.0, 0.0] ("ADC value") w116] -> w22
            frame False {
            }
            frame True {
              # "Corrected"
              # "Decode data, skipping first 4 lines"
              n53 = while {
                tunnel: w117 -> [w121]
                tunnel: [w130] -> w116 mode=indexing
                shift-right: [w125] -> _
                shift-left: _ -> [w126]
                i -> [w122]
                stop <- w129 continue-if-true
                # "Start at 4th line for ADCs"
                n54 = Increment(x=w122) -> (x+1=w119:i32)
                n55 = Increment(x=w119) -> (x+1=w123:i32)
                n56 = Increment(x=w123) -> (x+1=w120:i32)
                n57 = Increment(x=w120) -> (x+1=w124:i32)
                n58 = Increment(x=w124) -> (x+1=w132:i32)
                n59 = Pick Line(multi-line string=w121, line index=w124) -> (output string=w133:string)  [unwired: 1 in]
                n60 = Pick Line(multi-line string=w121, line index=w132) -> (output string=w131:string)  [unwired: 1 in]
                n61 = Scan From String "Scan From String"(input string=w133, initial scan location=0, error in=w126) -> (error out=w125:errorcluster, output 1=w130:dbl)  [unwired: 2 in, 2 out]
                "ADC Voltage Chart" <- w130
                n62 = String Length(string=w131) -> (length=w128:i32)
                n63 = Greater?(x=w128, y=1) -> (0:w129:bool)
              }
            }
          }
          "ADC value" <- w22
          n64 = case shown="True" w21 {
            tunnel: [w96 w109] -> w37
            tunnel: [w96 w108] -> w36
            tunnel: [w96 w104] -> w31
            tunnel: w23 -> [_ w100]
            tunnel: [FALSE w97] -> w20
            frame False {
              w96 = 0.0
            }
            frame True {
              w112 = 0
              n65 = Pick Line(multi-line string=w100, line index=1) -> (output string=w114:string)  [unwired: 1 in]
              n66 = Pick Line(multi-line string=w100, line index=0) -> (output string=w103:string)  [unwired: 1 in]
              n67 = Pick Line(multi-line string=w100, line index=2) -> (output string=w107:string)  [unwired: 1 in]
              n68 = Pick Line(multi-line string=w100, line index=3) -> (output string=w113:string)  [unwired: 1 in]
              n69 = Scan From String "Scan From String"(input string=w114, initial scan location=w112) -> (output 1=w109:dbl)  [unwired: 3 in, 3 out]
              "Frequency" <- w109
              n70 = Scan From String "Scan From String"(input string=w103, initial scan location=0) -> (output 1=w99:dbl)  [unwired: 3 in, 3 out]
              n71 = Scan From String "Scan From String"(input string=w107, initial scan location=0) -> (output 1=w104:dbl)  [unwired: 3 in, 3 out]
              "Amplitude" <- w104
              n72 = Scan From String "Scan From String"(input string=w113, initial scan location=w112) -> (output 1=w108:dbl)  [unwired: 3 in, 3 out]
              "Area" <- w108
              n73 = Greater?(x=w99, y=1.0) -> (0:w97:bool)
            }
          }
          "Fit OK" <- w20
          n74 = global write "Global 2.vi" "Fit OK"(w20) -> ()
        }
        frame #1 {
          # "Update peak center and area"
          n75 = global read "Global 2.vi" "UsePython"() -> (w137:bool)
          n76 = Replace Array Subset(array=w142, new element=w143, index=17) -> (w141:dbl[])
          n77 = Select(t=w140, s=w137, f="Quad sub area") -> (s? t:f=w139:dbl)
          n78 = Replace Array Subset(array=w141, new element=w149, index=19) -> (w151:dbl[])
          n79 = Multiply(x=w139, y=1000.0) -> (x*y=w146:dbl)
          n80 = Replace Array Subset(array=w151, new element=w146, index=11) -> (w150:dbl[])
          n81 = call-poly <vilib>:"Write To Spreadsheet File.vi"("transpose? (no:F)"=w152, "format (%.3f)"="%10.4f", "append to file? (new file:F)"=w153, "1D data"=w150, "file path (dialog if empty)"=w154) -> ()  [unwired: 3 in, 1 out]
        }
      }
    }
  }
